vi "IFwTest.vi"() -> ()   [LabVIEW 2017]
uses:
  <vilib>/Platform/TimedLoop/XDataNode/timing_clust.ctl
  <vilib>/Platform/TimedLoop/XDataNode/nitl_modes.ctl
  <vilib>/Platform/TimedLoop/XDataNode/wakeup.ctl
  <instrlib>/_niInstr/FIFO Register Bus/v1/FPGA/niInstr FIFO Register Bus v1 FPGA.lvclass
  C:/Program Files (x86)/National Instruments/LabVIEW 2017/instr.lib/_niInstr/Instruction Framework/v1/FPGA/Interfaces/Instruction Producer/Instruction Producer.lvclass
  <instrlib>/_niInstr/Instruction Framework/v1/FPGA/Helper Classes/Single Address Space Collection/Single Address Space Collection.lvclass
  C:/Program Files (x86)/National Instruments/LabVIEW 2017/instr.lib/_niInstr/Instruction Framework/v1/FPGA/Interfaces/Address Space Collection/Address Space Collection.lvclass
  <vilib>/rvi/Emulation/niFpgaGetClockAttributes.vi
  <vilib>/rvi/Emulation/niFpgaSctlEmulationGetInTimedLoop.vi
  <vilib>/rvi/Emulation/niFpgaEmulationReportErrorSimple.vi
  <vilib>/rvi/DataTransferAndStorage/Container/Common/niFpgaContainerExecOnDevCompGetState.vi
  <vilib>/rvi/Emulation/niFpgaEmulationIsFPGAContextNoSignature.vi
  <vilib>/rvi/DataTransferAndStorage/Container/Common/niFpgaContainerGetUniqueNameForEmu.vi
  <vilib>/rvi/Memory/Memory_Emulation/niFpgaMemoryEmulationCacheClearOnFirstRun.vi
  <vilib>/rvi/Memory/Memory_Emulation/nirvimemoryEmulationManagerCache_MakeExclusive.vi
  <vilib>/rvi/Memory/Memory_Emulation/niFpgaMemoryEmulationValidateCache.vi
  <vilib>/rvi/Memory/Memory_Emulation/nirvimemoryEmulationManagerCache_InsertValue.vi
  <vilib>/Utility/error.llb/Clear Errors.vi
  <vilib>/rvi/Memory/Memory_Emulation/nirvimemoryEmulationManagerCache_ReleaseExclusive.vi
  <vilib>/rvi/Memory/Memory_Emulation/nirvimemoryEmulationManagerCache_GetValue.vi
  <vilib>/rvi/Memory/Memory_Emulation/nirvimemoryEmulationManagerCache_SetValue.vi
  <vilib>/rvi/Emulation/niFpgaProcessEmulError.vi
  <vilib>/rvi/Emulation/niFpgaCriticalErrorInLSC.vi
  <vilib>/rvi/DataTransferAndStorage/Container/XNode/niFpgaContainer.xnode
  <vilib>/rvi/DataTransferAndStorage/Register/Emulation/niFpgaRegisterEmulationRefIn.vi
  <vilib>/Platform/TimedLoop/XDataNode/XDataNode.xnode
  AddressSpace.lvclass
  <instrlib>/_niInstr/Instruction Framework/v1/FPGA/Top Level Bus/Register Configuration/Register Configuration.lvclass
  <vilib>/Platform/TimedLoop/XDataNode/XDNodeRunTimeDep.lvlib
panel:
  out "HarmonicFilterEnable":bool
  out "HarmonicFilter":cluster{"ak":sgl, "bk":sgl}
  out "adjustTheta":sgl
  in  "detectedFreq":sgl
  out "dT":sgl
  out "lockDuration":u32
  out "expectedFreq":sgl
  out "freqBoundary":sgl
  in  "locked":bool
  out "reset":bool
  out "PLLRange":T1
  out "PLLGains":T2
  in  "fifo reg bus ctrl 0":u32
  out "fifo reg bus status 0":u32
  out "fifo reg bus data 0":u64
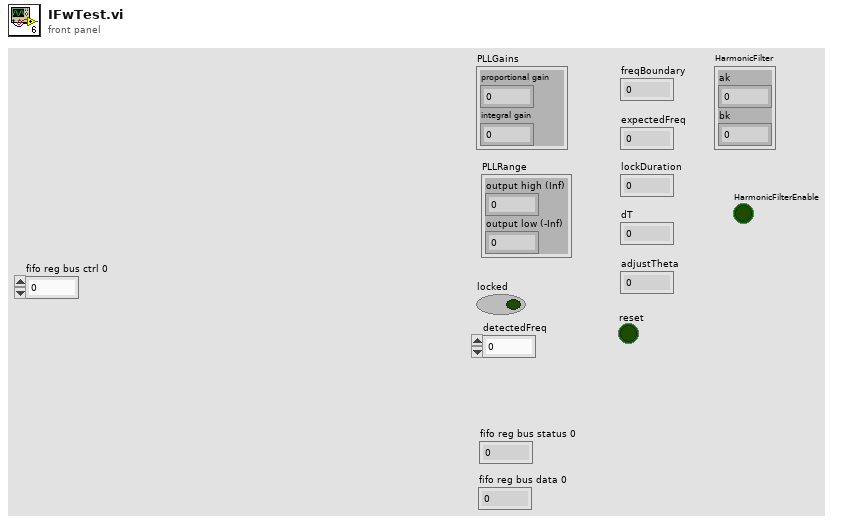
[diagram p1: front panel]
types:
  T1 = cluster{"output high (Inf)":sgl, "output low (-Inf)":sgl}
  T2 = cluster{"proportional gain":sgl, "integral gain":sgl}
  T3 = typedef "ThreePhasePLL.lvlib/registers.ctl" = cluster{"PLLGains":refnum<k21>, "PLLRange":refnum<k21>, "PLL_reset":refnum<k21>, "PLL_locked":refnum<k21>, "freqBoundaries":refnum<k21>, "expectedFreq":refnum<k21>, "lockDuration":refnum<k21>, "dT":refnum<k21>, "detectedFreq":refnum<k21>, "adjustTheta":refnum<k21>, "HarmonicFilter":refnum<k21>, "HarmonicFilterEnable":refnum<k21>}
  T4 = typedef "XDNodeRunTimeDep.lvlib/timing_clust.ctl" = cluster{"Expected End [f-1]":u64, "Actual End [f-1]":u64, "Finished Late? [f-1]":bool, "Expected End [i-1]":u64, "Actual End [i-1]":u64, "Finished Late? [i-1]":bool, "Expected Start [i]":u64, "Actual Start [i]":u64, "Expected Start [f]":u64, "Actual Start [f]":u64, "Source Name":string, "Structure Name":string, "Period":i64, "Deadline":i64, "Offset":i64, "Start":i64, "Priority":i32, "Timeout":i32, "Mode":T5, "Wakeup Reason":T6, "Error":errorcluster, "Source Type":string, "Secondary Source Type":string, "Global End Time":u64, "Global Start Time":u64, "Frame Duration":u64, "Iteration Duration":u64, "Assigned CPU":i32, "I/O Scan Engine Mode":u32}
  T5 = typedef "XDNodeRunTimeDep.lvlib/nitl_modes.ctl" = enum32{"No Change", "Process missed periods, maintain original phase", "Discard missed periods, maintain original phase", "Process missed periods, ignore original phase", "Discard missed periods, ignore original phase"}
  T6 = typedef "XDNodeRunTimeDep.lvlib/wakeup.ctl" = enum32{"Normal", "Aborted", "Asynchronous wakeup", "Timing source error", "Timed loop error", "Timeout"}
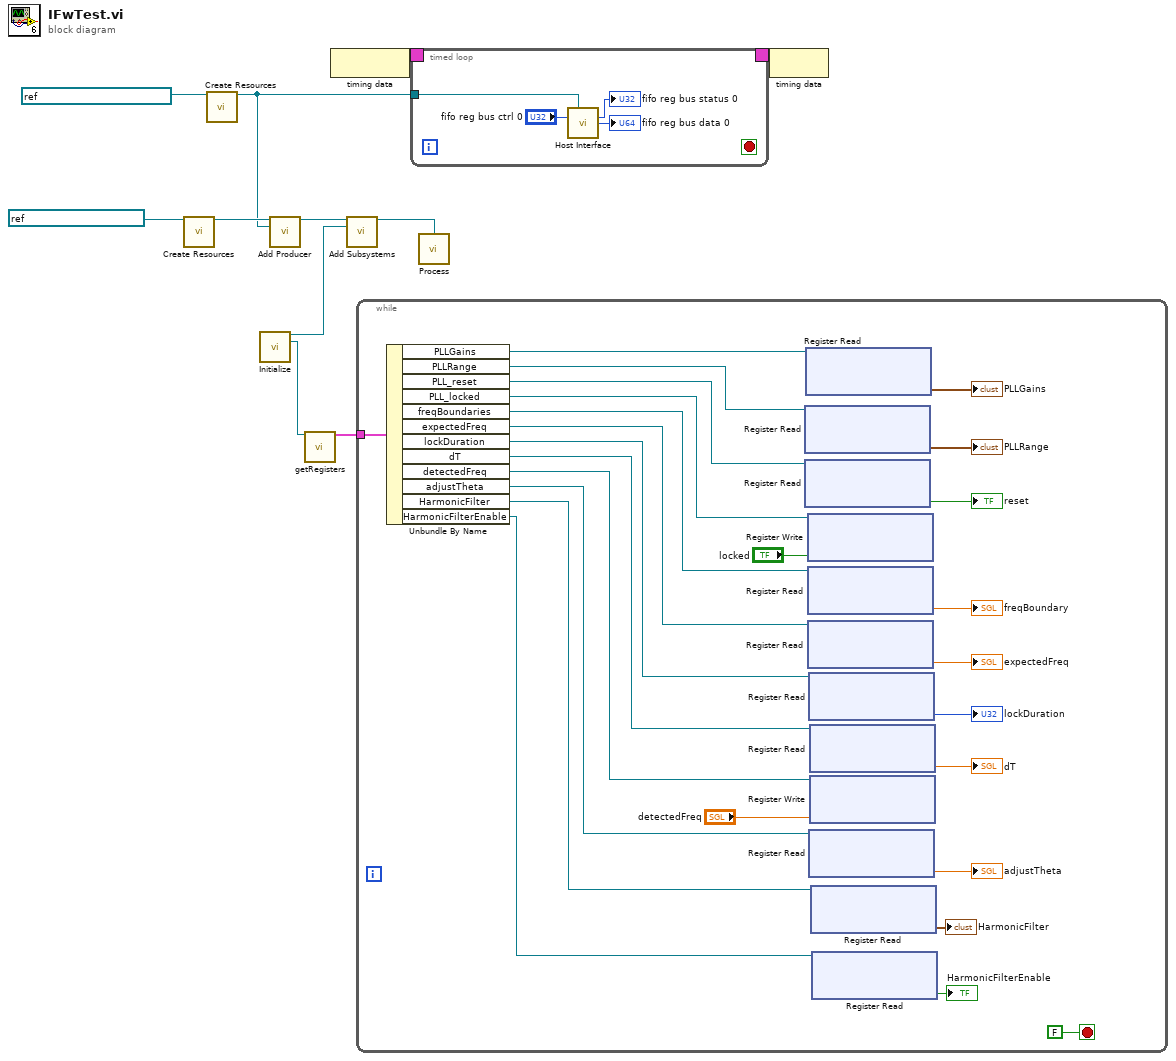
[diagram p0: block diagram]
diagram:
  n1 = call <instrlib>:"Create Resources.vi"("register clock"=refnum<k21> "40 MHz Onboard Clock") -> ("register configuration"=w7:refnum<class "Register Configuration.lvclass">)  [unwired: 14 in]
  n2 = call <instrlib>:"Create Resources.vi"("instruction fifo"=refnum<k21> "reg.host instruction fifo 0") -> ("fifo register bus"=w5:refnum<class "niInstr FIFO Register Bus v1 FPGA.lvclass">)  [unwired: 14 in]
  n3 = call "Initialize.vi"() -> ("subsysytem"=w3:refnum<class "Single Address Space Collection.lvclass">, "AddressSpace"=w2:refnum<class "AddressSpace.lvclass">)  [unwired: 14 in]
  n4 = call <instrlib>:"Add Producer.vi"("register configuration in"=w7, "instruction producer"=w5) -> ("register configuration out"=w6:refnum<class "Register Configuration.lvclass">)  [unwired: 13 in]
  n5 = call "getRegisters.vi"("AddressSpace"=w2) -> ("registers"=w1:T3)  [unwired: 14 in]
  n6 = node-c288() -> (w11:T4)
  n7 = call <instrlib>:"Add Subsystems.vi"("register configuration in"=w6, "subsystems"=w3) -> ("register configuration out"=w4:refnum<class "Register Configuration.lvclass">)  [unwired: 13 in]
  n8 = while {
    tunnel: w1 -> [w37]
    stop <- FALSE stop-if-true
    n9 = Unbundle By Name(w37) -> ("PLLGains"=w36:refnum<k21>, "PLLRange"=w35:refnum<k21>, "PLL_reset"=w34:refnum<k21>, "PLL_locked"=w33:refnum<k21>, "freqBoundaries"=w32:refnum<k21>, "expectedFreq"=w31:refnum<k21>, "lockDuration"=w30:refnum<k21>, "dT"=w29:refnum<k21>, "detectedFreq"=w28:refnum<k21>, "adjustTheta"=w27:refnum<k21>, "HarmonicFilter"=w16:refnum<k21>, "HarmonicFilterEnable"=w14:refnum<k21>)
    n10 = xnode "Register Read"("Register In"=w35) -> ("Data"=→"PLLRange":T1)  [unwired: 1 out]
    n11 = xnode "Register Read"("Register In"=w34) -> ("Data"=→"reset":bool)  [unwired: 1 out]
    n12 = xnode "Register Read"("Register In"=w36) -> ("Data"=→"PLLGains":T2)  [unwired: 1 out]
    n13 = xnode "Register Write"("Data"="locked", "Register In"=w33) -> ()  [unwired: 1 out]
    n14 = xnode "Register Read"("Register In"=w32) -> ("Data"=→"freqBoundary":sgl)  [unwired: 1 out]
    n15 = xnode "Register Read"("Register In"=w31) -> ("Data"=→"expectedFreq":sgl)  [unwired: 1 out]
    n16 = xnode "Register Read"("Register In"=w30) -> ("Data"=→"lockDuration":u32)  [unwired: 1 out]
    n17 = xnode "Register Read"("Register In"=w27) -> ("Data"=→"adjustTheta":sgl)  [unwired: 1 out]
    n18 = xnode "Register Read"("Register In"=w29) -> ("Data"=→"dT":sgl)  [unwired: 1 out]
    n19 = xnode "Register Write"("Data"="detectedFreq", "Register In"=w28) -> ()  [unwired: 1 out]
    n20 = xnode "Register Read"("Register In"=w16) -> ("Data"=→"HarmonicFilter":cluster{"ak":sgl, "bk":sgl})  [unwired: 1 out]
    n21 = xnode "Register Read"("Register In"=w14) -> ("Data"=→"HarmonicFilterEnable":bool)  [unwired: 1 out]
  }
  n22 = timed-loop {
    timing: w11 -> [_]
    timing-out: [_] -> w10
    tunnel: w5 -> [w41]
    stop <- _ stop-if-true
    n23 = call <instrlib>:"Host Interface.vi"("fifo register bus"=w41, "fifo reg bus ctrl 0"="fifo reg bus ctrl 0") -> ("fifo reg bus status 0"=→"fifo reg bus status 0":u32, "fifo reg bus data 0"=→"fifo reg bus data 0":u64)  [unwired: 12 in]
  }
  n24 = call <instrlib>:"Process.vi"("register configuration"=w4) -> ()  [unwired: 15 in]
  n25 = node-c288(w10) -> ()
